vi "Set Serial Settings.vi"(4 "Wire Mode":i16(ring)=-1 items=["Unknown"=-1, "RS485/Wire4"=0, "RS485/Wire2-EchoDTR"=1, "RS485/Wire2-CtrlDTR"=2, "RS485/Wire2-Auto"=3, "RS232/DTE"=128, "RS232/DCE"=129, "RS232/AUTO"=130], 5 "serial type":T2, 6 "parity (even)":T1=2 items=["None", "Odd", "Even", "Mark", "Space"], 7 "flow control (none)":T3 items=["None", "XON/XOFF", "RTS/CTS", "XON/XOFF & RTS/CTS", "DTR/DSR", "XON/XOFF & DTR/DSR"], 8 "error in (no error)":errorcluster, 9 "baud rate":u32=9600, 10 "VISA resource name":refnum<visa-resource-name>, 11 "Item Ref in":T4 format="%.0x") -> (0 "error out":errorcluster, 3 "Item Ref out":T4 format="%.0x")   [LabVIEW 2021, in "Modbus Master System Explorer.lvlib"]
uses:
  Modbus Master System Explorer.lvlib
  <vilib>/NI VeriStand/Custom Device API/Custom Device Item Ref.ctl
  Shared/Controls/Flow Control.ctl
  Shared/Controls/Serial Type.ctl
  Shared/Controls/Parity.ctl
  Shared/Constants.vi
  <vilib>/NI VeriStand/Custom Device API/Set Item Property (String).vi
  <vilib>/NI VeriStand/Custom Device API/Set Item Property (U32).vi
  <vilib>/NI VeriStand/Custom Device API/Set Item Property (U16).vi
  <vilib>/NI VeriStand/Custom Device API/Set Item Property (I32).vi
  <vilib>/NI VeriStand/Custom Device API/Custom Device API.lvlib
  Shared/Modbus Master Shared.lvlib
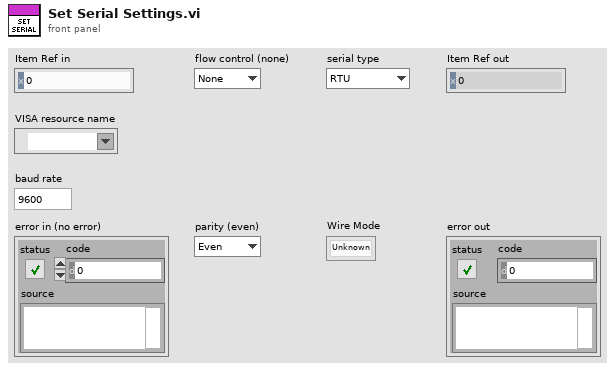
[diagram p1: front panel]
types:
  T1 = typedef "Modbus Master Shared.lvlib/Parity.ctl" = u16
  T2 = typedef "Modbus Master Shared.lvlib/Serial Type.ctl" = enum16{"RTU", "ASCII"}
  T3 = typedef "Modbus Master Shared.lvlib/Flow Control.ctl" = u16
  T4 = typedef "Custom Device API.lvlib/Custom Device Item Ref.ctl" = u64
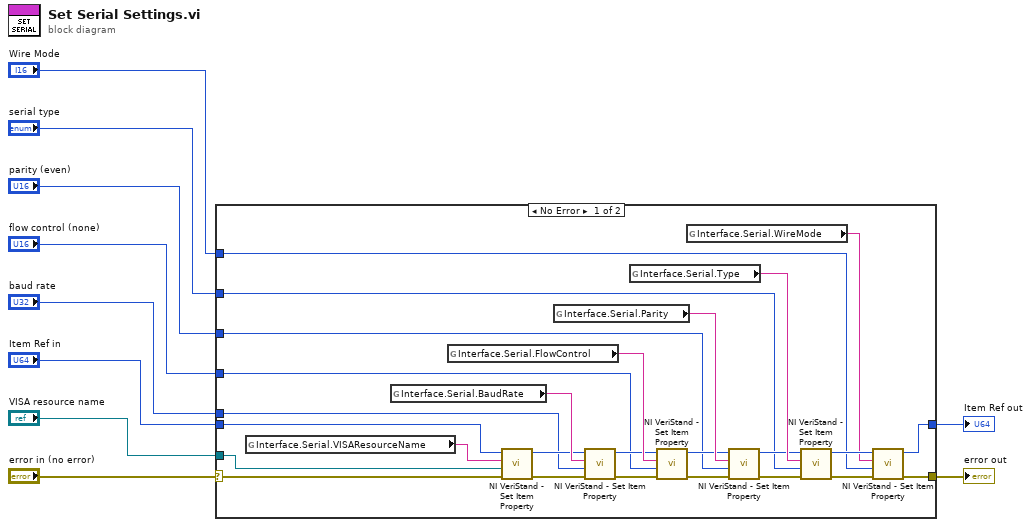
[diagram p0: block diagram]
diagram:
  n1 = case shown="No Error" "error in (no error)" {
    selector: "error in (no error)" -> [w24 w37]
    tunnel: [w14 w37] -> w10
    tunnel: [w13 w38] -> w9
    tunnel: "Item Ref in" -> [w23 w38]
    tunnel: "VISA resource name" -> [w22 _]
    tunnel: "baud rate" -> [w21 _]
    tunnel: "flow control (none)" -> [w20 _]
    tunnel: "parity (even)" -> [w19 _]
    tunnel: "serial type" -> [w18 _]
    tunnel: "Wire Mode" -> [w11 _]
    frame No Error {
      n2 = global read "Constants.vi" "Interface.Serial.VISAResourceName"() -> (w17:string)
      n3 = global read "Constants.vi" "Interface.Serial.BaudRate"() -> (w27:string)
      n4 = global read "Constants.vi" "Interface.Serial.FlowControl"() -> (w30:string)
      n5 = call-poly <vilib>:"NI VeriStand - Set Item Property.vi"("error in (no error)"=w24, "Value"=w22, "Property Name"=w17, "Item Ref in"=w23) -> ("error out"=w25:errorcluster, "Item Ref out"=w26:T4)  [unwired: 5 in, 1 out]
      n6 = global read "Constants.vi" "Interface.Serial.Parity"() -> (w33:string)
      n7 = call-poly <vilib>:"NI VeriStand - Set Item Property.vi"("error in (no error)"=w25, "Value"=w21, "Property Name"=w27, "Item Ref in"=w26) -> ("error out"=w28:errorcluster, "Item Ref out"=w29:T4)  [unwired: 5 in, 1 out]
      n8 = global read "Constants.vi" "Interface.Serial.Type"() -> (w36:string)
      n9 = call-poly <vilib>:"NI VeriStand - Set Item Property.vi"("error in (no error)"=w28, "Value"=w20, "Property Name"=w30, "Item Ref in"=w29) -> ("error out"=w31:errorcluster, "Item Ref out"=w32:T4)  [unwired: 5 in, 1 out]
      n10 = global read "Constants.vi" "Interface.Serial.WireMode"() -> (w12:string)
      n11 = call-poly <vilib>:"NI VeriStand - Set Item Property.vi"("error in (no error)"=w31, "Value"=w19, "Property Name"=w33, "Item Ref in"=w32) -> ("error out"=w34:errorcluster, "Item Ref out"=w35:T4)  [unwired: 5 in, 1 out]
      n12 = call-poly <vilib>:"NI VeriStand - Set Item Property.vi"("error in (no error)"=w34, "Value"=w18, "Property Name"=w36, "Item Ref in"=w35) -> ("error out"=w15:errorcluster, "Item Ref out"=w16:T4)  [unwired: 5 in, 1 out]
      n13 = call-poly <vilib>:"NI VeriStand - Set Item Property.vi"("error in (no error)"=w15, "Value"=w11, "Property Name"=w12, "Item Ref in"=w16) -> ("error out"=w14:errorcluster, "Item Ref out"=w13:T4)  [unwired: 5 in, 1 out]
    }
    frame Error {
    }
  }
  "error out" <- w10
  "Item Ref out" <- w9
